vi "RoundTripTest.vi"(8 "error in (no error)":errorcluster, 10 "Variant":variant, 11 "TestCase in":refnum<class "Python Data Tools Tests.lvclass">) -> (0 "error out":errorcluster, 2 "Python String":string, 3 "TestCase out":refnum<class "Python Data Tools Tests.lvclass">)   [LabVIEW 2020, in "Python Data Tools Tests.lvclass"]
uses:
  Python Data Tools Tests.lvclass
  Python Data Tools Tests.lvclass/Python Data Tools Tests.ctl
  source/jki_python_data_tools.lvlib
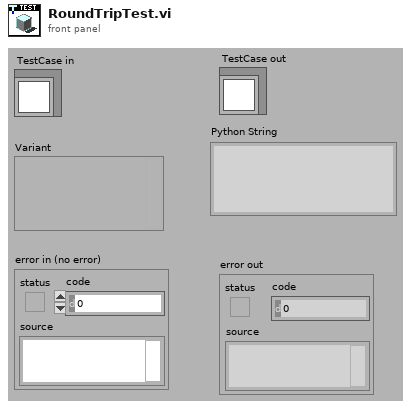
[diagram p1: front panel]
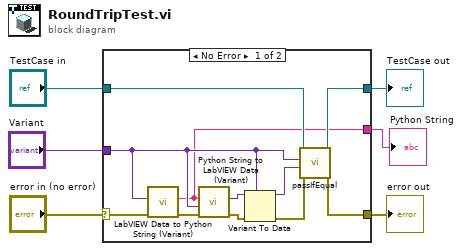
[diagram p0: block diagram]
diagram:
  n1 = case shown="No Error" "error in (no error)" {
    selector: "error in (no error)" -> [w8 w19]
    tunnel: "TestCase in" -> [w17 w18]
    tunnel: [w16 w18] -> w3
    tunnel: [w15 w19] -> w4
    tunnel: "Variant" -> [w9 _]
    tunnel: [w7 _] -> w1
    frame No Error {
      n2 = call "LabVIEW Data to Python String (Variant).vi"("error in (no error)"=w8, "LabVIEW Data"=w9) -> ("error out"=w14:errorcluster, "Python String"=w7:string)  [unwired: 8 in]
      n3 = call "Python String to LabVIEW Data (Variant).vi"("error in (no error)"=w14, "type"=w9, "Python String"=w7) -> ("error out"=w12:errorcluster, "LabVIEW Data"=w13:variant)  [unwired: 7 in]
      n4 = Variant To Data(error in=w12, type=w9, Variant=w13) -> (data=w10:variant, error out=w11:errorcluster)
      n5 = call-dynamic "passIfEqual.vi"("error in (no error)"=w11, "y"=w10, "x"=w9, "TestCase in"=w17) -> ("error out"=w15:errorcluster, "TestCase out"=w16:refnum<class "Python Data Tools Tests.lvclass">)  [unwired: 6 in]
    }
    frame Error {
    }
  }
  "error out" <- w4
  "TestCase out" <- w3
  "Python String" <- w1
